vi "Teleop.vi"(10 "Match Info":T1={"Autonomous Elapsed Seconds"=0.0, "TeleOp Elapsed Seconds"=0.0, "Disabled Elapsed Seconds"=0.0, "Visited Autonomous"=FALSE, "Visited TeleOp"=FALSE, "Visited Disabled"=FALSE, "Autonomous Settings"={"Autonomous Style"=enum."Independent", "VI Refnum"=refnum}}, 11 "Call Context":T2) -> ()   [LabVIEW 2015]
doc: "This VI is called for each enabled TeleOp packet received from the DS. It is typically used to read from joysticks and other inputs and update I/O or setpoints for timed control loops. It should complete and return within 20 milliseconds or risk missing DS packets."
uses:
  <vilib>/Rock Robotics/WPI/DriverStation/WPI_DriverStationDerivedRobotMode.ctl
  <vilib>/Rock Robotics/WPI/DriverStation/WPI_DriverStationMatch Info.ctl
  Gear/Implementation/Gear.ctl
  Drive/Implementation/Global Drive Variables.vi
  <vilib>/Rock Robotics/Network Tables/NT Write Boolean Array.vi
  <vilib>/Rock Robotics/Network Tables/NT Write Numeric Array.vi
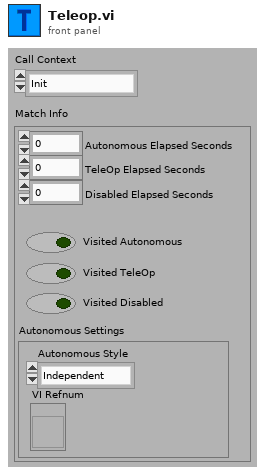
[diagram p1: front panel]
types:
  T1 = typedef "WPI_DriverStationMatch Info.ctl" = cluster{"Autonomous Elapsed Seconds":dbl, "TeleOp Elapsed Seconds":dbl, "Disabled Elapsed Seconds":dbl, "Visited Autonomous":bool, "Visited TeleOp":bool, "Visited Disabled":bool, "Autonomous Settings":cluster{"Autonomous Style":enum16{"Iterative", "Independent"}, "VI Refnum":refnum<vi>}}
  T2 = typedef "WPI_DriverStationDerivedRobotMode.ctl" = enum16{"Init", "Execute", "Stop"}
  T3 = typedef "Gear.ctl" = enum16{"High", "Low"}
  T4 = typedef "JoystickData.ctl" = cluster{"Axes":dbl[], "Buttons":bool[]}
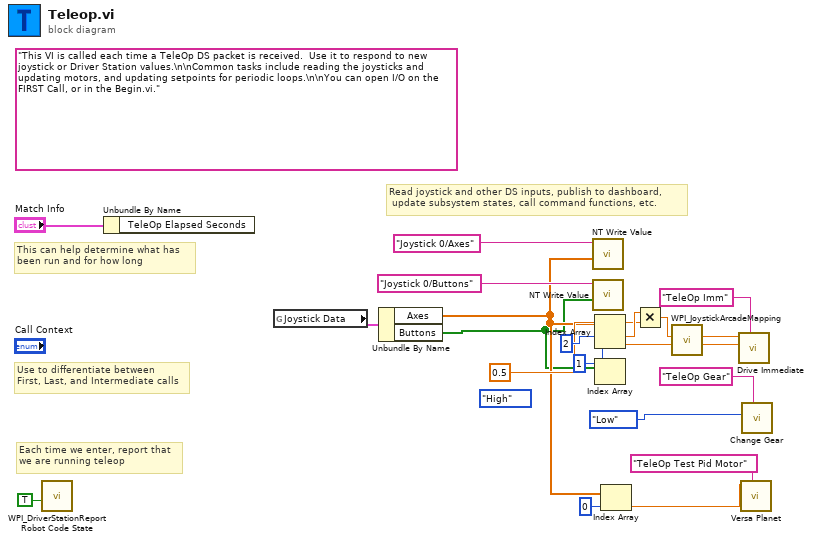
[diagram p0: block diagram]
diagram:
  (unwired) Gear."High" ("Gear")
  (unwired) "This VI is called each time a TeleOp DS packet is received.  Use it to respond to new joystick or Driver Station values.\n\nCommon tasks include reading the joysticks and updating motors, and updating setpoints for periodic loops.\n\nYou can open I/O on the FIRST Call, or in the Begin.vi."
  # "Read joystick and other DS inputs, publish to dashboard,\n update subsystem states, call command functions, etc."
  # "Each time we enter, report that\nwe are running teleop"
  # "Use to differentiate between\nFirst, Last, and Intermediate calls"
  # "This can help determine what has\nbeen run and for how long"
  n1 = call <vilib>:"WPI_DriverStationReport Robot Code State.vi"("TeleOp"=TRUE ("Autonomous")) -> ()  [unwired: 10 in, 1 out]
  n2 = Unbundle By Name("Match Info") -> ()  [unwired: 1 out]
  n3 = global read "Global Drive Variables.vi" "Joystick Data"() -> (w3:T4)
  n4 = Unbundle By Name(w3) -> ("Axes"=w2:dbl[], "Buttons"=w1:bool[])
  n5 = call-poly <vilib>:"NT Write Value.vi"("Numeric Array"=w2, "Name"="Joystick 0/Axes") -> ()  [unwired: 9 in, 1 out]
  n6 = call-poly <vilib>:"NT Write Value.vi"("Boolean Array"=w1, "Name"="Joystick 0/Buttons") -> ()  [unwired: 9 in, 1 out]
  n7 = Index Array(array=w2, index #1=2 ("index"), index #2=1 ("index")) -> (element #1=w6:dbl, element #2=w18:dbl)
  n8 = Index Array(array=w1) -> ()  [unwired: 1 in, 1 out]
  n9 = Index Array(array=w2, index=0) -> (element=w10:dbl)
  n10 = Multiply(x=w6, y=0.5) -> (x*y=w5:dbl)
  n11 = call <vilib>:"WPI_JoystickArcadeMapping.vi"("Y axis value"=w18, "X axis value"=w5) -> ("Right Motor Value"=w14:dbl, "Left Motor Value"=w15:dbl)  [unwired: 8 in]
  n12 = call "Drive Immediate.vi"("Description"="TeleOp Imm", "Right Setpoint"=w14, "Left Setpoint"=w15) -> ()  [unwired: 8 in, 1 out]
  n13 = call "Versa Planet.vi"("Description"="TeleOp Test Pid Motor", "Setpoint"=w10) -> ()  [unwired: 10 in]
  n14 = call "Change Gear.vi"("Description"="TeleOp Gear", "Gear"=Gear."Low") -> ()  [unwired: 10 in]
